vi "[FGV]ColorMatch_Template.vi"(7 "CMTemplateCommand":string, 8 "error in (no error)":errorcluster, 10 "Image Name Array":string[](array[string]), 11 "Image Array":T1[](array[typedef])) -> (0 "error out":errorcluster, 2 "Image Name Array 2":string[](array[string]), 3 "Image Array 2":T1[](array[typedef]))   [LabVIEW 2019]
uses:
  <vilib>/vision/Image Controls.llb/IMAQ Image.ctl
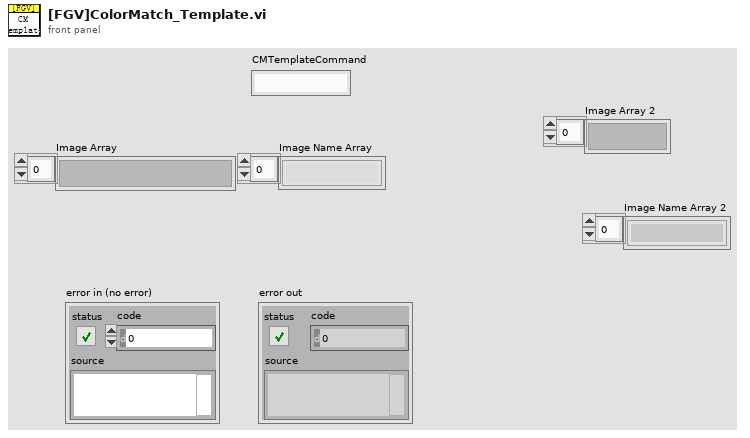
[diagram p1: front panel]
types:
  T1 = typedef "IMAQ Image.ctl" = refnum<image>
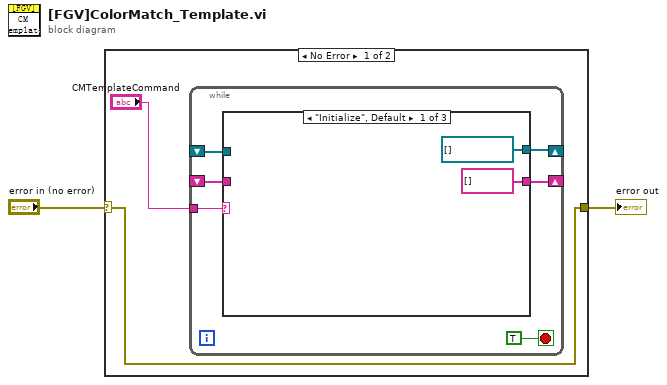
[diagram p0: block diagram]
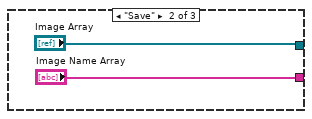
[diagram p2: hidden frame]
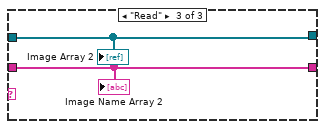
[diagram p3: hidden frame]
diagram:
  n1 = case shown="No Error" "error in (no error)" {
    selector: "error in (no error)" -> [w4 w17]
    tunnel: [w4 w17] -> w1
    frame No Error {
      n2 = while {
        shift-right: [w9] -> _
        shift-left: _ -> [w8]
        shift-right: [w7] -> _
        shift-left: _ -> [w6]
        tunnel: "CMTemplateCommand" -> [w5]
        stop <- TRUE stop-if-true
        n3 = case shown="\"Initialize\", Default" w5 {
          tunnel: [T1[] [] ("Image Array") "Image Array" w16] -> w9
          tunnel: w8 -> [_ _ w16]
          tunnel: [string[] [] ("Image Name Array") "Image Name Array" w15] -> w7
          tunnel: w6 -> [_ _ w15]
          frame "Initialize", Default {
          }
          frame "Save" {
          }
          frame "Read" {
            "Image Array 2" <- w16
            "Image Name Array 2" <- w15
          }
        }
      }
    }
    frame Error {
    }
  }
  "error out" <- w1
